vi "DWF FGEN Configure Arbitrary Waveform Gain and Offset.vi"(0 "Instrument Handle In":u32, 7 "Gain":dbl=1.0 caption="Gain (no change)", 9 "DC Offset":dbl caption="DC Offset (no change)", 11 "Error In":errorcluster caption="Error In (no error)") -> (4 "Instrument Handle Out":u32, 15 "Error Out":errorcluster)   [LabVIEW 2015, in "DigilentWF.lvlib"]
doc: "Configures the instrument to output an arbitrary waveform with a specified gain and offset value. The waveform is output either after the end of the current waveform if output is enabled, or immediately after output is enabled. Any unwired configuration terminals do not change the existing values of those parameters."
uses:
  <vilib>/DigilentWF/DigilentWF.lvlib
  dwf.dll
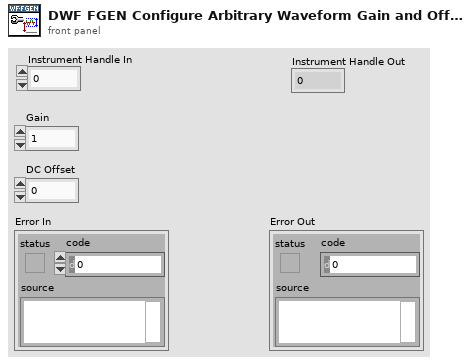
[diagram p1: front panel]
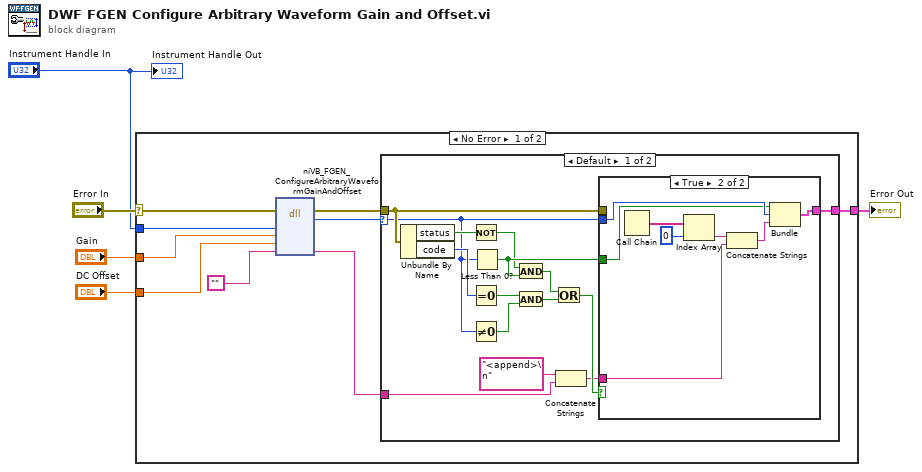
[diagram p0: block diagram]
diagram:
  n1 = case "outter_case" shown="No Error" "Error In" {
    selector: "Error In" -> [w13 w40]
    tunnel: [w14 w40] -> w4
    tunnel: "Instrument Handle In" -> [w11 _]
    tunnel: "Gain" -> [w10 _]
    tunnel: "DC Offset" -> [w9 _]
    frame No Error {
      n2 = dll-call lib="dwf.*" fn="niVB_FGEN_ConfigureArbitraryWaveformGainAndOffset"(error in=w13, "instrumentHandle"=w11, "gain"=w10, "dcOffset"=w9, "szError"="") -> (error out=w12:errorcluster, "return type"=w8:u32, "szError"=w6:string)  [unwired: 5 in, 1 out]
      n3 = case "inner_case" shown="Default" w8 {
        selector: w8 -> [w19 _]
        tunnel: w12 -> [w20 w39]
        tunnel: [w16 w39] -> w14
        tunnel: w6 -> [w15 _]
        frame Default {
          n4 = Unbundle By Name(w20) -> ("status"=w24:bool, "code"=w28:i32)
          n5 = Not(x=w24) -> (.not. x?=w27:bool)
          n6 = Equal To 0?(x=w28) -> (x = 0?=w23:bool)
          n7 = Not Equal To 0?(x=w19) -> (x != 0?=w26:bool)
          n8 = Less Than 0?(x=w19) -> (x < 0?=w29:bool)
          n9 = And(x=w27, y=w29) -> (x .and. y?=w25:bool)
          n10 = And(x=w23, y=w26) -> (x .and. y?=w22:bool)
          n11 = Or(x=w25, y=w22) -> (x .or. y?=w21:bool)
          n12 = Concatenate Strings("<append>\n" ("string"), w15) -> (w18:string)
          n13 = case shown="True" w21 {
            tunnel: [w30 w37] -> w16
            tunnel: w19 -> [_ w36]
            tunnel: w29 -> [_ w35]
            tunnel: w20 -> [w30 _]
            tunnel: w18 -> [_ w31]
            frame False {
            }
            frame True {
              n14 = Call Chain() -> (call chain=w34:string[])
              n15 = Index Array(array=w34, index=0) -> (element=w33:string)
              n16 = Concatenate Strings(w33, w31) -> (w38:string)
              n17 = Bundle(w35, "return type"=w36, w38) -> (w37:cluster{bool, "return type":u32, string})  [unwired: 1 out]
            }
          }
        }
        frame 0 {
        }
      }
    }
    frame Error {
    }
  }
  "Error Out" <- w4
  "Instrument Handle Out" <- "Instrument Handle In"
